vi "FTW-Benchmark-ActorThroughput.vi"() -> ()   [LabVIEW 2015]
uses:
  source/actor/Ether/FTW-Ether.lvclass
  source/actor/Connector/FTW-ActorConnector.lvclass
  <vilib>/ptbypt/NI_PtbyPt.lvlib
panel:
  in  "RT Stop Button":bool
  out "Roundtrip Time":dbl format="%.3psec"
  in  "Timeout":i32=1000
  in  "Connect to existing":bool
  in  "Connection":string(combo)="inproc://*"
  out "Throughput":cluster{dbl, "mean":dbl, dbl}(graph)
  in  "Response Payload Size":u32=1024
  in  "Message Payload Size":i32=1024
  out "Instance Inbox Address":string
  out "Initialized Response":string
  out "error out":errorcluster
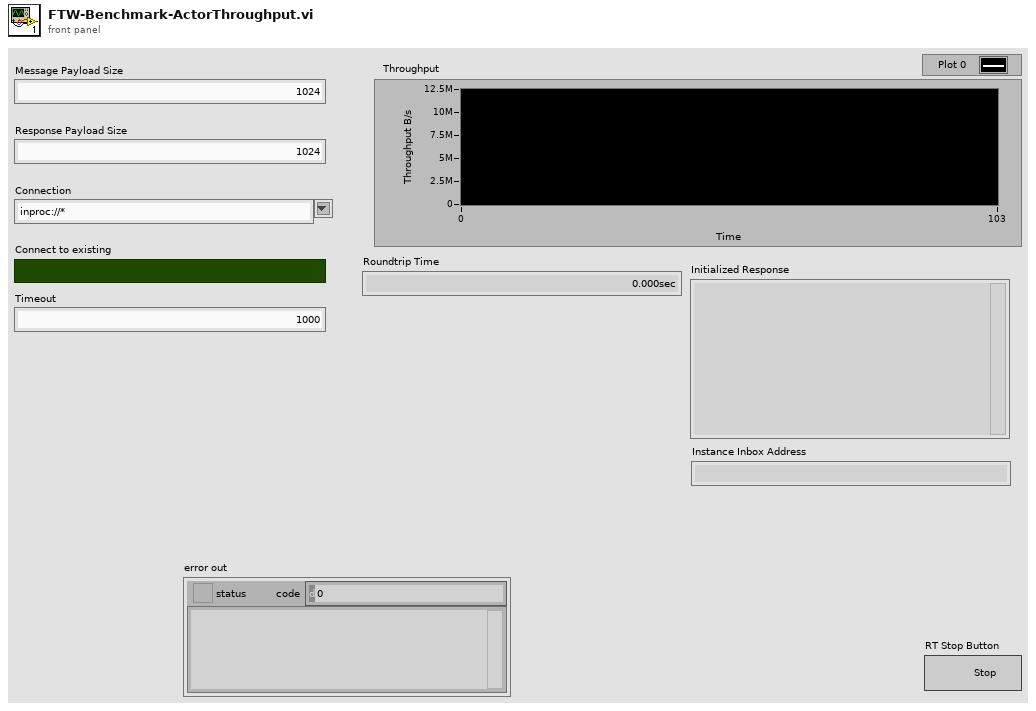
[diagram p1: front panel]
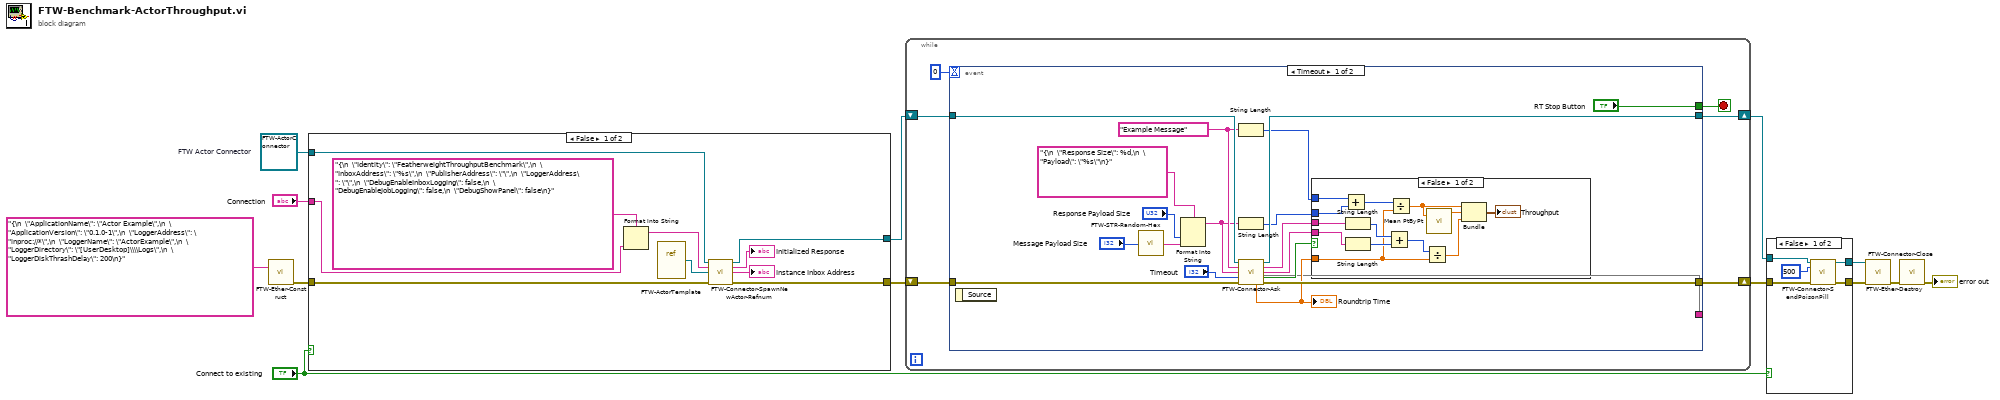
[diagram p0: block diagram]
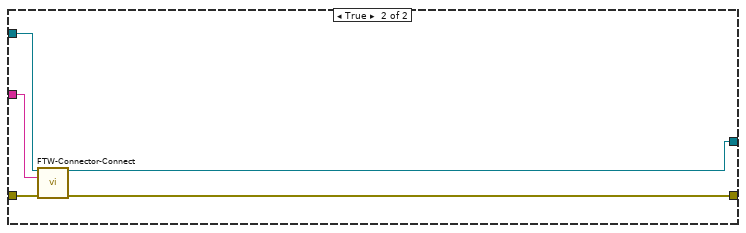
[diagram p3: hidden frame]
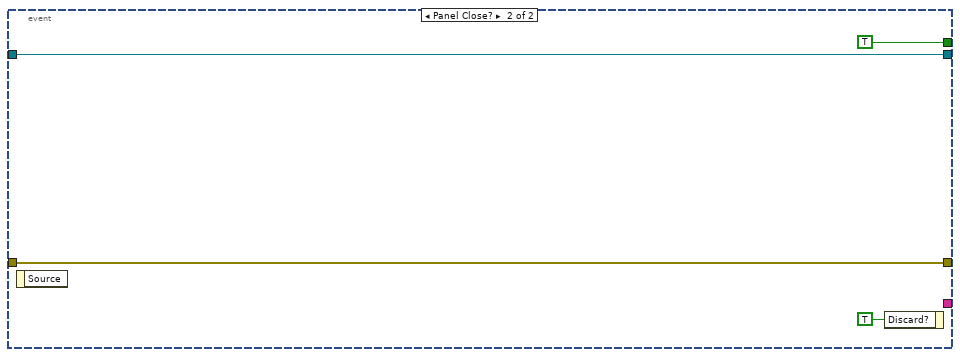
[diagram p5: hidden frame]
diagram:
  w2 = refnum<class "FTW-ActorConnector.lvclass"> refnum  # FTW Actor Connector
  n1 = call "FTW-Ether-Construct.vi"("FTW Ether Configuration"="{\n  \"ApplicationName\": \"Actor Example\",\n  \"ApplicationVersion\": \"0.1.0-1\",\n  \"LoggerAddress\": \"inproc://*\",\n  \"LoggerName\": \"ActorExample\",\n  \"LoggerDirectory\": \"[UserDesktop]\\\\Logs\",\n  \"LoggerDiskThrashDelay\": 200\n}") -> ("error out"=w13:errorcluster)  [unwired: 14 in]
  n2 = case shown="False" "Connect to existing" {
    tunnel: w13 -> [w23 w28]
    tunnel: [w20 w26] -> w9
    tunnel: [w19 w27] -> w8
    tunnel: "Connection" -> [w16 w25]
    tunnel: w2 -> [w15 w24]
    frame False {
      n3 = Format Into String(format string="{\n  \"Identity\": \"FeatherweightThroughputBenchmark\",\n  \"InboxAddress\": \"%s\",\n  \"PublisherAddress\": \"\",\n  \"LoggerAddress\": \"\",\n  \"DebugEnableInboxLogging\": false,\n  \"DebugEnableJobLogging\": false,\n  \"DebugShowPanel\": false\n}" ("Actor 1 Configuration"), w16) -> (resulting string=w17:string)  [unwired: 2 in, 1 out]
      n4 = vi-ref "FTW-ActorTemplate.vi"() -> (w14:refnum<vi>)
      n5 = call "FTW-Connector-SpawnNewActor-Refnum.vi"("FTW Actor Connector Type"=w15, "Configuration"=w17, "Actor VI Refnum"=w14, "error in"=w23) -> ("FTW Actor Connector"=w20:refnum<class "FTW-ActorConnector.lvclass">, "Initialized Response"=→"Initialized Response":string, "Instance Inbox Address"=→"Instance Inbox Address":string, "error out"=w19:errorcluster)  [unwired: 8 in]
    }
    frame True {
      n6 = call-dynamic "FTW-Connector-Connect.vi"("FTW Actor Connector Type"=w24, "Instance Inbox Address"=w25, "error in"=w28) -> ("FTW Actor Connector"=w26:refnum<class "FTW-ActorConnector.lvclass">, "error out"=w27:errorcluster)  [unwired: 11 in]
    }
  }
  n7 = while {
    shift-right: [w32] -> w7
    shift-left: w9 -> [w34]
    shift-right: [w31] -> w6
    shift-left: w8 -> [w33]
    stop <- w30 stop-if-true
    n8 = event shown="[0] Timeout" {
      selector: _ -> [_ _]
      dyn-events: _ -> [_ _]
      timeout: 0 -> [_ _]
      tunnel: w34 -> [w53 w68]
      tunnel: w33 -> [w52 w69]
      tunnel: [w51 w68] -> w32
      tunnel: [w50 w69] -> w31
      tunnel: ["RT Stop Button" TRUE] -> w30
      tunnel: [w35 _] -> _
      event Timeout {
        w44 = "Example Message" ("Request Header")
        n9 = event-data() -> ()  [unwired: 1 in, 1 out]
        n10 = call "FTW-STR-Random-Hex.vi"("String Length"="Message Payload Size") -> ("Random Hex String"=w46:string)  [unwired: 3 in]
        n11 = Format Into String(format string="{\n  \"Response Size\": %d,\n  \"Payload\": \"%s\"\n}" ("Request Body"), "Response Payload Size", w46) -> (resulting string=w43:string)  [unwired: 2 in, 1 out]
        n12 = String Length(string=w44) -> (length=w42:i32)
        n13 = String Length(string=w43) -> (length=w41:i32)
        n14 = call "FTW-Connector-Ask.vi"("FTW Actor Connector"=w53, "Request Header"=w44, "Request Body"=w43, "Timeout"="Timeout", "error in"=w52) -> ("FTW Actor Connector out"=w51:refnum<class "FTW-ActorConnector.lvclass">, "Response Header"=w40:string, "Response Body"=w39:string, "Timed out?"=w37:bool, 13:w35, "Roundtrip Time"=w38:dbl, "error out"=w50:errorcluster)  [unwired: 4 in]
        "Roundtrip Time" <- w38
        n15 = case shown="False" w37 {
          tunnel: w42 -> [w66 _]
          tunnel: w41 -> [w65 _]
          tunnel: w40 -> [w59 _]
          tunnel: w39 -> [w58 _]
          tunnel: w38 -> [w57 _]
          frame False {
            n16 = Add(x=w66, y=w65) -> (x+y=w64:i32)
            n17 = String Length(string=w59) -> (length=w60:i32)
            n18 = String Length(string=w58) -> (length=w61:i32)
            n19 = Add(x=w60, y=w61) -> (x+y=w62:i32)
            n20 = Divide(x=w64, y=w57) -> (x/y=w55:dbl)
            n21 = Divide(x=w62, y=w57) -> (x/y=w56:dbl)
            n22 = call <vilib>:"Mean PtByPt.vi"("x"=w55) -> ("mean"=w54:dbl)  [unwired: 3 in, 1 out]
            n23 = Bundle(w55, "mean"=w54, w56) -> (→"Throughput":cluster{dbl, "mean":dbl, dbl})  [unwired: 1 in]
          }
          frame True {
          }
        }
      }
      event Panel Close? {
        n24 = event-data() -> ()  [unwired: 1 in, 1 out]
        n25 = event-data("Discard?"=TRUE) -> ()  [unwired: 1 in, 1 out]
      }
    }
  }
  n26 = case shown="False" "Connect to existing" {
    tunnel: w7 -> [w75 w77]
    tunnel: w6 -> [w74 w76]
    tunnel: [w73 w77] -> w5
    tunnel: [w72 w76] -> w4
    frame False {
      n27 = call-dynamic "FTW-Connector-SendPoisonPill.vi"("FTW Actor Connector"=w75, "Timeout"=500, "error in"=w74) -> ("FTW Actor Connector out"=w73:refnum<class "FTW-ActorConnector.lvclass">, "error out"=w72:errorcluster)  [unwired: 7 in, 4 out]
    }
    frame True {
    }
  }
  n28 = call-dynamic "FTW-Connector-Close.vi"("FTW Actor Connector"=w5, "error in"=w4) -> ("error out"=w10:errorcluster)  [unwired: 13 in]
  n29 = call "FTW-Ether-Destroy.vi"("error in"=w10) -> ("error out"=→"error out":errorcluster)  [unwired: 14 in]
